vi "Test App Owned Process Context is Set.vi"(8 "error in (no error)":errorcluster, 11 "Application Test in":refnum<class "Application Dev Test.lvclass">) -> (0 "error out":errorcluster, 3 "Application Test out":refnum<class "Application Dev Test.lvclass">)   [LabVIEW 2020, in "Application Dev Test.lvclass"]
uses:
  Application Dev Test.lvclass
  C:/Program Files (x86)/National Instruments/LabVIEW 2020/vi.lib/Astemes/LUnit/Test Case.lvclass
  source/Framework/Process/Process.lvclass
  source/Framework/Process/Process.lvclass/Process.ctl
  source/Framework/Application/Application.lvclass/Application.ctl
  <vilib>/Astemes/LUnit/Test Case.lvclass/Test Case.ctl
  <vilib>/Astemes/LUnit/LUnit Assertion Result.lvclass/LUnit Assertion Result.ctl
  <vilib>/Astemes/LUnit/LUnit Test Case Result.lvclass/LUnit Test Case Result.ctl
  <vilib>/Astemes/LUnit/LUnit Method Result.lvclass/LUnit Method Result.ctl
  source/Framework/Application/Private/Add Process to Map.vi
  source/Framework/Application/Private/Start Idle Processes if Running.vi
  source/Framework/Application/Private/Throw Error If Process Already in App.vi
  source/Framework/Process/Protected/Messaging/Enqueue Message.vi
  source/Framework/Process/Public/Lifecycle/Get Lifecycle State.vi
  source/Framework/Process/Protected/SubVIs/Set Context.vi
  source/Framework/Application/Private/Retrieve Process from App.vi
  source/Framework/Application/Private/Parse Process Name.vi
  source/Framework/Application/Private/Get Process from Map.vi
  <vilib>/Astemes/LUnit/Palette/Pass If Equal.vi/cbf50e99-f124-4847-863a-8e9794d3dede.vi
  source/Framework/Process/Private/SubVIs/Wait for finish.vi
  source/Framework/Process/Private/SubVIs/Set Lifecycle State.vi
  source/Framework/Process/Private/SubVIs/Handle Debug Data.vi
  <vilib>/Utility/error.llb/Clear Errors.vi
  source/Framework/Process/Public/Lifecycle/Leave Process Loop.vi
  source/Framework/Process/Protected/Messaging/Request Message.vi
  <vilib>/AdvancedString/Delimited String to 1D String Array.vi
  <vilib>/Astemes/LUnit/Palette/Pass.vi
  <vilib>/Astemes/LUnit/Palette/Fail.vi
  <vilib>/Astemes/LUnit/Compare Variants.vi
  <vilib>/Astemes/LUnit/Describe Comparison.vi
  <vilib>/Astemes/LUnit/Set Assertion Type.vi
  source/Framework/Logging/Log Debug.vi
  <vilib>/AdvancedString/1D String Array to Delimited String.vi
  <vilib>/Utility/High Resolution Relative Seconds.vi
  source/Framework/Process/Private/SubVIs/Enqueue Request Message.vi
  <vilib>/Astemes/LUnit/Add test result.vi
  <vilib>/Astemes/LUnit/LUnit Write Passed.vi
  <vilib>/Astemes/LUnit/LUnit Write Message.vi
  <vilib>/Astemes/LUnit/LUnit Write Description.vi
  <vilib>/Astemes/LUnit/Variant to string.vi
  <vilib>/Astemes/LUnit/LUnit Write Assertion Type.vi
  <vilib>/Astemes/LUnit/LUnit Record Assertion Result.vi
  <vilib>/Astemes/LUnit/LUnit Aggregate Assertion Results.vi
  <vilib>/Astemes/LUnit/Assertion Result/LUnit Read Status.vi
  <vilib>/Astemes/LUnit/LUnit Read Message.vi
  <vilib>/Astemes/LUnit/LUnit Read Description.vi
  <vilib>/Astemes/LUnit/Method Result/LUnit Merge Status.vi
  <vilib>/Astemes/LUnit/LUnit Concatenate result strings.vi
  source/Framework/Application/Application.lvclass
  C:/Git/astemes-triarc-framework/source/Framework/Process/Process.lvclass
  <vilib>/Utility/error.llb/Error Cluster From Error Code.vi
  source/Framework/Process/Private/SubVIs/Wait for Response Message.vi
  <vilib>/Utility/Data Type/Get Type Information.vi
  <vilib>/Utility/LVClass/Get LV Class Name.vi
  <vilib>/Astemes/LUnit/LUnit Assertion Result.lvclass
  <vilib>/Astemes/LUnit/Test Case.lvclass
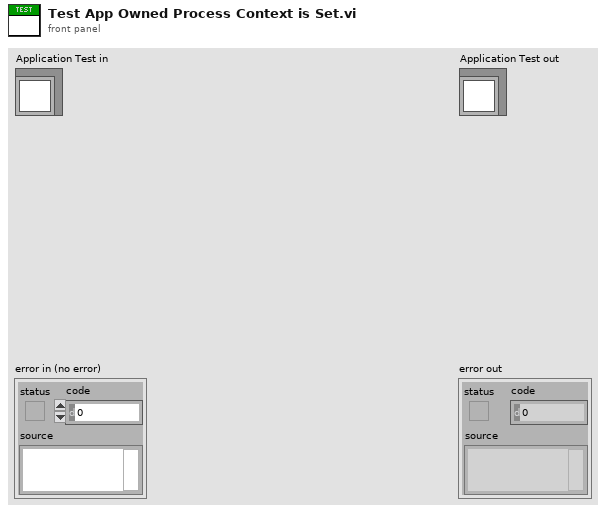
[diagram p1: front panel]
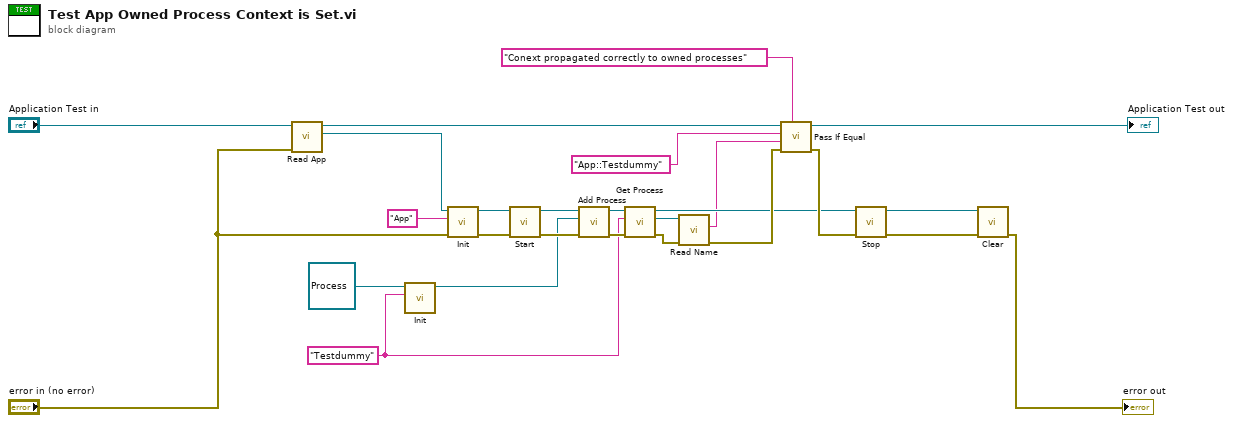
[diagram p0: block diagram]
diagram:
  w13 = "Testdummy" ("Name")
  n1 = call "Read App.vi"("error in (no error)"="error in (no error)", "Application Test In"="Application Test in") -> ("App out"=w25:refnum<class "Application.lvclass">, "Application Test Out"=w26:refnum<class "Application Dev Test.lvclass">)  [unwired: 7 in, 1 out]
  n2 = call-dynamic "Init.vi"("Name"=w13, "Process In"=refnum<class "Process.lvclass"> refnum) -> ("Process Out"=w17:refnum<class "Process.lvclass">)  [unwired: 8 in, 1 out]
  n3 = call-dynamic "Init.vi"("error in (no error)"="error in (no error)", "Name"="App", "Process In"=w25) -> ("error out"=w23:errorcluster, "Process Out"=w24:refnum<class "Application.lvclass">)  [unwired: 7 in]
  n4 = call "Start.vi"("error in (no error)"=w23, "Process In"=w24) -> ("error out"=w20:errorcluster, "Process Out"=w11:refnum<class "Application.lvclass">)  [unwired: 7 in, 1 out]
  n5 = call "Add Process.vi"("error in (no error)"=w20, "Process"=w17, "Application In"=w11) -> ("error out"=w21:errorcluster, "Application Out"=w4:refnum<class "Application.lvclass">)  [unwired: 7 in]
  n6 = call "Get Process.vi"("error in (no error)"=w21, "Process Name"=w13, "Application In"=w4) -> ("error out"=w9:errorcluster, "App Process"=w10:refnum<class "Process.lvclass">, "Application Out"=w7:refnum<class "Application.lvclass">)  [unwired: 6 in]
  n7 = call "Read Name.vi"("error in (no error)"=w9, "Process In"=w10) -> ("error out"=w8:errorcluster, "Qualified Name"=w1:string)  [unwired: 6 in, 2 out]
  n8 = call <vilib>:"Pass If Equal.vi"("Description"="Conext propagated correctly to owned processes", "error in (no error)"=w8, "Actual"=w1, "Expected"="App::Testdummy", "LUnit Test Case In"=w26) -> ("error out"=w18:errorcluster, "LUnit Test Case Out"=→"Application Test out":refnum<class "Application Dev Test.lvclass">)  [unwired: 5 in]
  n9 = call "Stop.vi"("error in (no error)"=w18, "Process In"=w7) -> ("error out"=w14:errorcluster, "Process Out"=w22:refnum<class "Application.lvclass">)  [unwired: 7 in, 1 out]
  n10 = call-dynamic "Clear.vi"("error in (no error)"=w14, "Application In"=w22) -> ("error out"=→"error out":errorcluster)  [unwired: 9 in]
